vi "Downlink MICS.vi"(8 "Error In":errorcluster, 10 "Downlink":u8[][](array[numeric]) format="%02x", 11 "Reference In":i32) -> (0 "Error Out":errorcluster, 3 "Reference Out":i32)   [LabVIEW 2009]
uses:
  Reference.vi
panel:
  # "DOWNLINK"
  # "Block 1"
  # "Block 2"
  # "Block 3"
  # "Block 4"
  # "b1"
  # "b2"
  # "b3"
  # "b4"
  # "b5"
  # "b6"
  # "b7"
  # "b8"
  # "b9"
  # "b10"
  # "b11"
  # "b12"
  # "b13"
  # "b14"
  # "b15"
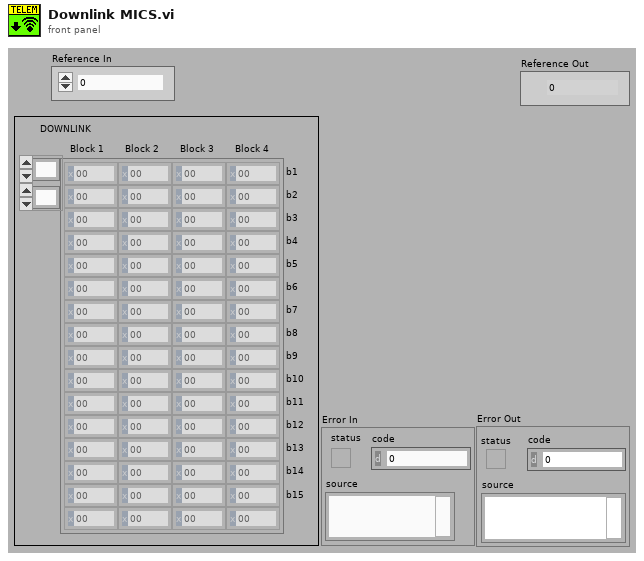
[diagram p1: front panel]
types:
  T1 = cluster{"[0]":i32, "[1]":i32, "[2]":i32, "[3]":i32, "[4]":i32, "[5]":i32, "[6]":i32, "[7]":i32, "[8]":i32}
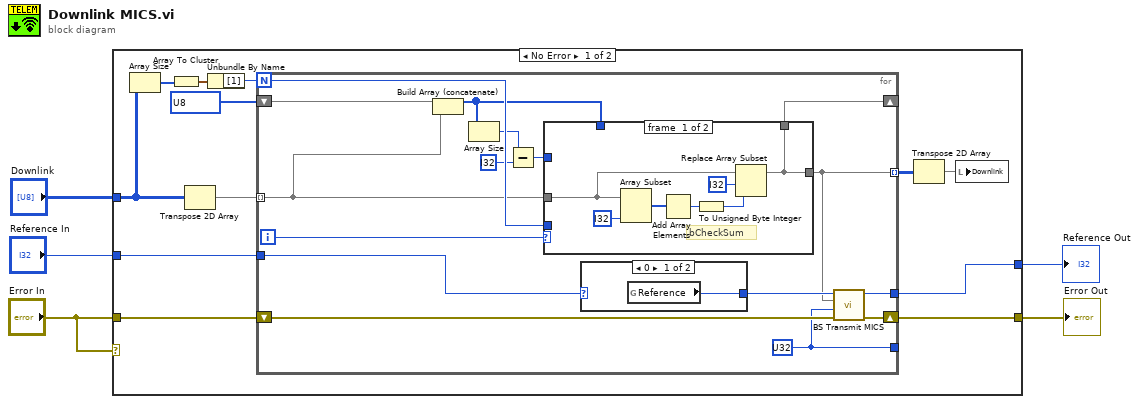
[diagram p0: block diagram]
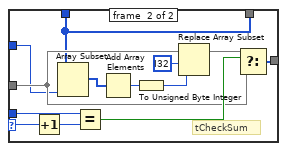
[diagram p2: hidden frame]
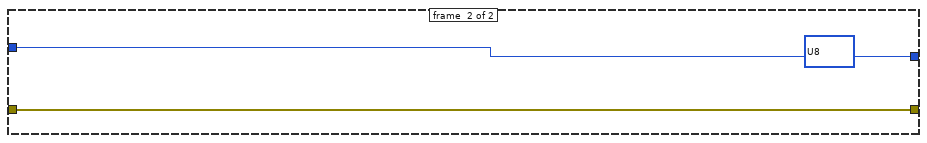
[diagram p4: hidden frame]
diagram:
  n1 = case shown="No Error" "Error In" {
    tunnel: "Downlink" -> [w14 _]
    tunnel: "Error In" -> [w13 w57]
    tunnel: "Reference In" -> [w12 w56]
    tunnel: [w7 w57] -> w3
    tunnel: [w8 w56] -> w1
    frame #0 {
      n2 = Array Size(array=w14) -> (size(s)=w17:i32[])
      n3 = Array To Cluster(array=w17) -> (cluster=w16:T1)
      n4 = Transpose 2D Array(2D array=w14) -> (transposed array=w11:u8[][])
      n5 = Unbundle By Name(w16) -> ("[1]"=w15:i32)
      n6 = for {
        N: w15 -> [w28]
        tunnel: w11 -> [w20] mode=indexing
        shift-right: [w32] -> w7
        shift-left: w13 -> [w33]
        tunnel: w12 -> [w30]
        tunnel: [w29] -> w8
        tunnel: [w27] -> _
        tunnel: [w26] -> w10 mode=indexing
        shift-right: [w18] -> _
        shift-left: u8[] ? -> [w25]
        i -> [w21]
        w27 = u32 ? ("nBytes")
        n7 = Build Array (concatenate)(w25, w20) -> (w19:u8[])
        n8 = Array Size(array=w19) -> (size(s)=w24:i32)
        n9 = Subtract(x=w24, y=i32 ?) -> (x-y=w22:i32)
        n10 = case shown="1, Default" w21 {
          selector: w21 -> [_ w50]
          tunnel: w20 -> [w39 w46]
          tunnel: [w34 w47] -> w26
          tunnel: w28 -> [_ w51]
          tunnel: w19 -> [_ w41]
          tunnel: w22 -> [_ w45]
          tunnel: [w34 w41] -> w18
          frame #0 {
            # "bCheckSum"
            n11 = Array Subset(array=w39, length=i32 ?) -> (w37:u8[])  [unwired: 1 in]
            n12 = Add Array Elements(numeric array=w37) -> (sum=w36:u8)
            n13 = To Unsigned Byte Integer(number=w36) -> (unsigned 8bit integer=w35:u8)
            n14 = Replace Array Subset(array=w39, new element=w35, index=i32 ?) -> (w34:u8[])
          }
          frame #1 {
            # "tCheckSum"
            n15 = Increment(x=w50) -> (x+1=w52:i32)
            n16 = Array Subset(array=w41, length=w45) -> (w43:u8[])  [unwired: 1 in]
            n17 = Equal?(x=w51, y=w52) -> (x = y?=w49:bool)
            n18 = Add Array Elements(numeric array=w43) -> (sum=w44:u8)
            n19 = To Unsigned Byte Integer(number=w44) -> (unsigned 8bit integer=w42:u8)
            n20 = Replace Array Subset(array=w46, new element=w42, index=i32 ?) -> (w48:u8[])
            n21 = Select(t=w48, s=w49, f=w46) -> (s? t:f=w47:u8[])
          }
        }
        n22 = case shown="0" w30 {
          selector: w30 -> [_ w55]
          tunnel: [w54 w55] -> w31
          frame #0 {
            n23 = global read "Reference.vi" "Reference"() -> (w54:i32)
          }
          frame #1 {
          }
        }
        n24 = call <vilib>:"BS Transmit MICS.vi"("Error In"=w33, "nBytes"=w27, "data"=w26, "Reference In"=w31) -> ("Error Out"=w32:errorcluster, "Reference Out"=w29:i32)  [unwired: 4 in]
      }
      n25 = Transpose 2D Array(2D array=w10) -> (transposed array=w9:u8[][])
      n26 = local write "Downlink"(w9) -> ()
    }
    frame #1 {
      (unwired) u8[][] ? ("buf")
    }
  }
  "Error Out" <- w3
  "Reference Out" <- w1
